vi "result_display.vi"(7 "note count":i32, 8 "lvl info":T1, 9 "score info":T2, 10 "timer":u32, 11 "new picture in":picture) -> (3 "new picture":picture)   [LabVIEW 2023]
uses:
  <vilib>/picture/picture.llb/Draw True-Color Pixmap.vi
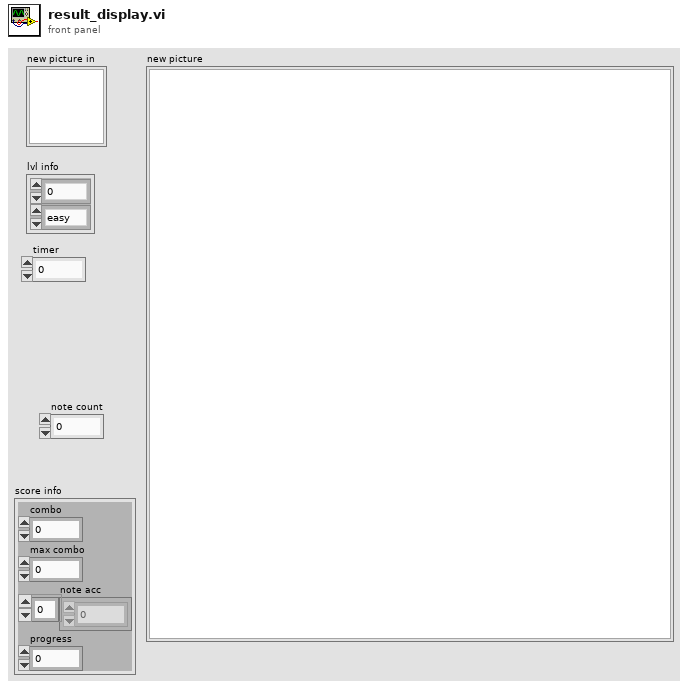
[diagram p1: front panel]
types:
  T1 = cluster{enum16{"0", "1"}, enum16{"easy", "hard"}}
  T2 = cluster{"combo":i32, "max combo":i32, "note acc":i32[], "progress":dbl}
  T3 = cluster{"horizontal":enum16{"left", "center", "right"}, "vertical":enum16{"top", "center", "bottom"}}
  T4 = cluster{"Font Name:":string, "Size":i16, "Strikeout?":bool, "Italic?":bool, "Underline?":bool, "Outline?":bool, "Shadow?":bool, "Bold?":bool}
  T5 = cluster{"Width":i16, "Style":enum32{"Solid", "Dash", "Dot", "DashDot", "DashDotDot"}}
  T6 = enum16{"User-specified Font", "Application Font", "System Font", "Dialog Font"}
  T7 = typedef "imagedata.ctl" = cluster{"image type":i32, "image depth":i32, "image":u8[], "mask":u8[], "colors":u32[], "Rectangle":cluster{"left":i16, "top":i16, "right":i16, "bottom":i16}}
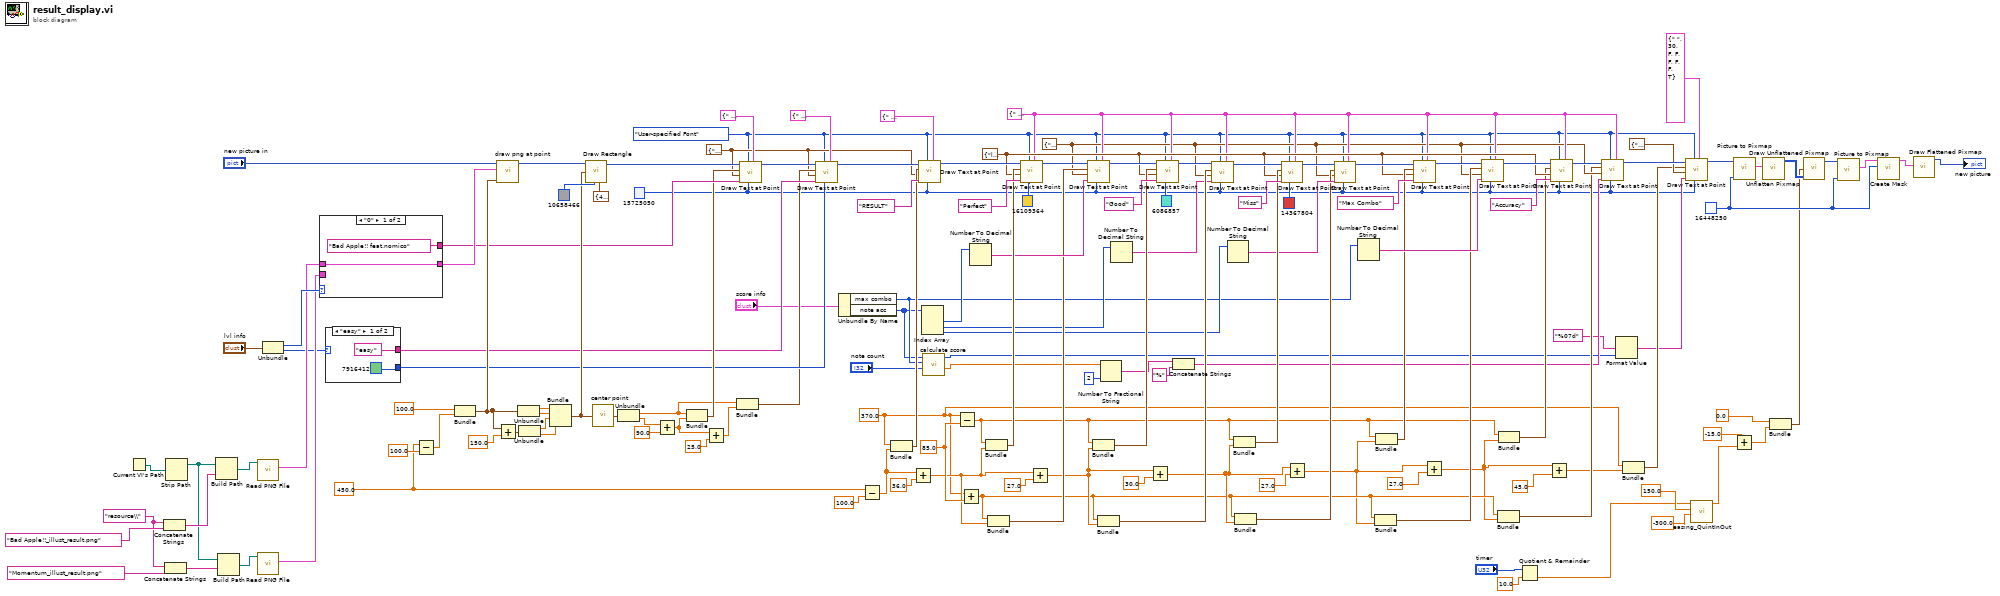
[diagram p0: block diagram]
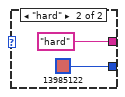
[diagram p2: hidden frame]
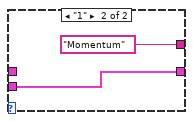
[diagram p3: hidden frame]
diagram:
  w11 = u32 16448250 ("color(black)")
  (unwired) 27.0
  w42 = T3 {"horizontal"=enum."right", "vertical"=enum."center"} ("alignment(left, top)")
  w50 = T3 {"horizontal"=enum."left", "vertical"=enum."center"} ("alignment(left, top)")
  w81 = 85.0
  w43 = T4 {"Font Name:"=" ", "Size"=20, "Strikeout?"=FALSE, "Italic?"=FALSE, "Underline?"=FALSE, "Outline?"=FALSE, "Shadow?"=FALSE, "Bold?"=TRUE} ("[user-specified font]")
  w125 = 450.0
  w20 = u32 15725050 ("text color(black)")
  w31 = 370.0
  w91 = T3 {"horizontal"=enum."center", "vertical"=enum."center"} ("alignment(left, top)")
  w27 = T6."User-specified Font" ("desired font(Application)")
  w142 = "resource\\"
  n1 = Current VI's Path() -> (path=w144:path)
  n2 = Concatenate Strings(w142, "Bad Apple!!_illust_result.png") -> (w140:string)
  n3 = Concatenate Strings(w142, "Momentum_illust_result.png") -> (w138:string)
  n4 = Strip Path(path=w144) -> (stripped path=w139:path)  [unwired: 1 out]
  n5 = Build Path(base path=w139, name or relative path=w140) -> (appended path=w137:path)
  n6 = Build Path(base path=w139, name or relative path=w138) -> (appended path=w136:path)
  n7 = call <vilib>:"Read PNG File.vi"("path to PNG file"=w137) -> ("image data"=w130:T7)  [unwired: 8 in, 2 out]
  n8 = call <vilib>:"Read PNG File.vi"("path to PNG file"=w136) -> ("image data"=w129:T7)  [unwired: 8 in, 2 out]
  n9 = Unbundle("lvl info") -> (w131:enum16{"0", "1"}, w104:enum16{"easy", "hard"})
  n10 = case shown="\"0\"" w131 {
    tunnel: w130 -> [w146 _]
    tunnel: w129 -> [_ w148]
    tunnel: [w146 w148] -> w127
    tunnel: ["Bad Apple!! feat.nomico" "Momentum"] -> w110
    frame "0" {
    }
    frame "1" {
    }
  }
  n11 = case shown="\"easy\"" w104 {
    tunnel: ["easy" "hard"] -> w100
    tunnel: [u32 7916412 ("color(black)") u32 13985122 ("color(black)")] -> w99
    frame "easy" {
    }
    frame "hard" {
    }
  }
  n12 = Subtract(x=w125, y=100.0) -> (x-y=w124:dbl)
  n13 = Bundle(100.0, w124) -> (w120:cluster{dbl, dbl})  [unwired: 1 in]
  n14 = call "draw png at point.vi"("top left point(0, 0)"=w120, "image data"=w127, "new picture in"="new picture in") -> ("new picture out"=w115:picture)  [unwired: 8 in]
  n15 = Add(x=w120, y=150.0) -> (x+y=w118:cluster{dbl, dbl})
  n16 = Unbundle(w120) -> (w122:dbl, w121:dbl)
  n17 = Unbundle(w118) -> (w117:dbl, w116:dbl)
  n18 = Bundle(w122, w121, w117, w116) -> (w112:cluster{dbl, dbl, dbl, dbl})  [unwired: 1 in]
  n19 = call <vilib>:"Draw Rectangle.vi"("picture"=w115, "rect"=w112, "color(black)"=u32 10658466, "pen"=T5 {"Width"=4, "Style"=enum."Solid"}) -> ("new picture"=w111:picture)  [unwired: 5 in]
  n20 = call "center point.vi"("border"=w112) -> ("center"=w108:cluster{dbl, dbl})  [unwired: 4 in]
  n21 = Unbundle(w108) -> (w98:dbl, w107:dbl)
  n22 = Add(x=w107, y=90.0) -> (x+y=w96:dbl)
  n23 = Bundle(w98, w96) -> (w105:cluster{dbl, dbl})  [unwired: 1 in]
  n24 = Add(x=w96, y=25.0) -> (x+y=w95:dbl)
  n25 = Bundle(w98, w95) -> (w94:cluster{dbl, dbl})  [unwired: 1 in]
  n26 = call <vilib>:"Draw Text at Point.vi"("[user-specified font]"=T4 {"Font Name:"=" ", "Size"=17, "Strikeout?"=FALSE, "Italic?"=FALSE, "Underline?"=FALSE, "Outline?"=FALSE, "Shadow?"=FALSE, "Bold?"=TRUE}, "text color(black)"=w20, "desired font(Application)"=w27, "text"=w110, "alignment(left, top)"=w91, "origin"=w105, "picture"=w111) -> ("new picture"=w103:picture)  [unwired: 3 in, 1 out]
  n27 = call <vilib>:"Draw Text at Point.vi"("[user-specified font]"=T4 {"Font Name:"=" ", "Size"=16, "Strikeout?"=FALSE, "Italic?"=FALSE, "Underline?"=FALSE, "Outline?"=FALSE, "Shadow?"=FALSE, "Bold?"=TRUE}, "text color(black)"=w99, "desired font(Application)"=w27, "text"=w100, "alignment(left, top)"=w91, "origin"=w94, "picture"=w103) -> ("new picture"=w101:picture)  [unwired: 3 in, 1 out]
  n28 = Unbundle By Name("score info") -> ("max combo"=w41:i32, "note acc"=w40:i32[])
  n29 = Subtract(x=w125, y=100.0) -> (x-y=w90:dbl)
  n30 = Bundle(w31, w90) -> (w133:cluster{dbl, dbl})  [unwired: 1 in]
  n31 = Add(x=w90, y=36.0) -> (x+y=w77:dbl)
  n32 = call <vilib>:"Draw Text at Point.vi"("[user-specified font]"=T4 {"Font Name:"=" ", "Size"=29, "Strikeout?"=FALSE, "Italic?"=FALSE, "Underline?"=FALSE, "Outline?"=FALSE, "Shadow?"=FALSE, "Bold?"=TRUE}, "text color(black)"=w20, "desired font(Application)"=w27, "text"="RESULT", "alignment(left, top)"=w91, "origin"=w133, "picture"=w101) -> ("new picture"=w93:picture)  [unwired: 3 in, 1 out]
  n33 = Index Array(array=w40) -> (element #1=w85:i32, element #2=w73:i32, element #3=w61:i32)  [unwired: 3 in]
  n34 = call "calculate score.vi"("note count"="note count", "max combo"=w41, "note acc"=w40) -> ("accuracy"=w36:dbl, "score"=w23:i32)  [unwired: 7 in]
  n35 = Subtract(x=w31, y=w81) -> (x-y=w49:dbl)
  n36 = Add(x=w31, y=w81) -> (x+y=w48:dbl)
  n37 = Number To Decimal String(number=w85) -> (decimal integer string=w84:string)  [unwired: 1 in]
  n38 = Bundle(w49, w77) -> (w88:cluster{dbl, dbl})  [unwired: 1 in]
  n39 = Bundle(w48, w77) -> (w82:cluster{dbl, dbl})  [unwired: 1 in]
  n40 = call <vilib>:"Draw Text at Point.vi"("[user-specified font]"=w43, "text color(black)"=u32 16109364, "desired font(Application)"=w27, "text"="Perfect", "alignment(left, top)"=w50, "origin"=w88, "picture"=w93) -> ("new picture"=w83:picture)  [unwired: 3 in, 1 out]
  n41 = Add(x=w77, y=27.0) -> (x+y=w66:dbl)
  n42 = call <vilib>:"Draw Text at Point.vi"("[user-specified font]"=w43, "text color(black)"=w20, "desired font(Application)"=w27, "text"=w84, "alignment(left, top)"=w42, "origin"=w82, "picture"=w83) -> ("new picture"=w80:picture)  [unwired: 3 in, 1 out]
  n43 = Bundle(w49, w66) -> (w75:cluster{dbl, dbl})  [unwired: 1 in]
  n44 = Bundle(w48, w66) -> (w74:cluster{dbl, dbl})  [unwired: 1 in]
  n45 = Number To Fractional String(number=w36, precision (6)=i16 2) -> (F-format string=w35:string)  [unwired: 2 in]
  n46 = Number To Decimal String(number=w73) -> (decimal integer string=w72:string)  [unwired: 1 in]
  n47 = Add(x=w66, y=30.0) -> (x+y=w55:dbl)
  n48 = call <vilib>:"Draw Text at Point.vi"("[user-specified font]"=w43, "text color(black)"=u32 6086857, "desired font(Application)"=w27, "text"="Good", "alignment(left, top)"=w50, "origin"=w75, "picture"=w80) -> ("new picture"=w71:picture)  [unwired: 3 in, 1 out]
  n49 = Concatenate Strings(w35, "%" ("string")) -> (w33:string)
  n50 = call <vilib>:"Draw Text at Point.vi"("[user-specified font]"=w43, "text color(black)"=w20, "desired font(Application)"=w27, "text"=w72, "alignment(left, top)"=w42, "origin"=w74, "picture"=w71) -> ("new picture"=w70:picture)  [unwired: 3 in, 1 out]
  n51 = Number To Decimal String(number=w61) -> (decimal integer string=w64:string)  [unwired: 1 in]
  n52 = Bundle(w49, w55) -> (w65:cluster{dbl, dbl})  [unwired: 1 in]
  n53 = Bundle(w48, w55) -> (w62:cluster{dbl, dbl})  [unwired: 1 in]
  n54 = call <vilib>:"Draw Text at Point.vi"("[user-specified font]"=w43, "text color(black)"=u32 14367804, "desired font(Application)"=w27, "text"="Miss", "alignment(left, top)"=w50, "origin"=w65, "picture"=w70) -> ("new picture"=w63:picture)  [unwired: 3 in, 1 out]
  n55 = Add(x=w55, y=27.0) -> (x+y=w47:dbl)
  n56 = call <vilib>:"Draw Text at Point.vi"("[user-specified font]"=w43, "text color(black)"=w20, "desired font(Application)"=w27, "text"=w64, "alignment(left, top)"=w42, "origin"=w62, "picture"=w63) -> ("new picture"=w60:picture)  [unwired: 3 in, 1 out]
  n57 = Number To Decimal String(number=w41) -> (decimal integer string=w57:string)  [unwired: 1 in]
  n58 = Bundle(w48, w47) -> (w53:cluster{dbl, dbl})  [unwired: 1 in]
  n59 = Bundle(w49, w47) -> (w54:cluster{dbl, dbl})  [unwired: 1 in]
  n60 = call <vilib>:"Draw Text at Point.vi"("[user-specified font]"=w43, "text color(black)"=w20, "desired font(Application)"=w27, "text"="Max Combo", "alignment(left, top)"=w50, "origin"=w54, "picture"=w60) -> ("new picture"=w58:picture)  [unwired: 3 in, 1 out]
  n61 = Add(x=w47, y=27.0) -> (x+y=w29:dbl)
  n62 = call <vilib>:"Draw Text at Point.vi"("[user-specified font]"=w43, "text color(black)"=w20, "desired font(Application)"=w27, "text"=w57, "alignment(left, top)"=w42, "origin"=w53, "picture"=w58) -> ("new picture"=w52:picture)  [unwired: 3 in, 1 out]
  n63 = Bundle(w48, w29) -> (w38:cluster{dbl, dbl})  [unwired: 1 in]
  n64 = Bundle(w49, w29) -> (w45:cluster{dbl, dbl})  [unwired: 1 in]
  n65 = Quotient & Remainder(x="timer", y=10.0 ("interval (10 ms)")) -> (floor(x/y)=w4:dbl)  [unwired: 1 out]
  n66 = Add(x=w29, y=45.0) -> (x+y=w28:dbl)
  n67 = call <vilib>:"Draw Text at Point.vi"("[user-specified font]"=w43, "text color(black)"=w20, "desired font(Application)"=w27, "text"="Accuracy", "alignment(left, top)"=w50, "origin"=w45, "picture"=w52) -> ("new picture"=w44:picture)  [unwired: 3 in, 1 out]
  n68 = call <vilib>:"Draw Text at Point.vi"("[user-specified font]"=w43, "text color(black)"=w20, "desired font(Application)"=w27, "text"=w33, "alignment(left, top)"=w42, "origin"=w38, "picture"=w44) -> ("new picture"=w32:picture)  [unwired: 3 in, 1 out]
  n69 = Format Value(format string="%07d", value (0)=w23) -> (output string=w21:string)  [unwired: 1 in]
  n70 = Bundle(w31, w28) -> (w24:cluster{dbl, dbl})  [unwired: 1 in]
  n71 = call <vilib>:"Draw Text at Point.vi"("[user-specified font]"=T4 {"Font Name:"=" ", "Size"=30, "Strikeout?"=FALSE, "Italic?"=FALSE, "Underline?"=FALSE, "Outline?"=FALSE, "Shadow?"=FALSE, "Bold?"=TRUE}, "text color(black)"=w20, "desired font(Application)"=w27, "text"=w21, "alignment(left, top)"=T3 {"horizontal"=enum."center", "vertical"=enum."center"}, "origin"=w24, "picture"=w32) -> ("new picture"=w16:picture)  [unwired: 3 in, 1 out]
  n72 = call "easing_QuintInOut.vi"("distance"=-300.0, "interval (10 ms)"=150.0, "time"=w4) -> ("current position"=w2:dbl)  [unwired: 8 in]
  n73 = Add(x=-15.0 ("interval (10 ms)"), y=w2) -> (x+y=w3:dbl)
  n74 = call <vilib>:"Picture to Pixmap.vi"("Background Color"=w11, "picture"=w16) -> ("image data"=w15:T7)  [unwired: 8 in, 1 out]
  n75 = call <vilib>:"Unflatten Pixmap.vi"("image data"=w15) -> ("24-bit pixmap"=w14:u32[][])  [unwired: 4 in, 6 out]
  n76 = Bundle("interval (10 ms)"=0.0, w3) -> (w7:cluster{"interval (10 ms)":dbl, dbl})  [unwired: 1 in]
  n77 = call-poly <vilib>:"Draw Unflattened Pixmap.vi"("top left point(0, 0)"=w7, "data (RGB format)"=w14) -> ("new picture"=w13:picture)  [unwired: 7 in]
  n78 = call <vilib>:"Picture to Pixmap.vi"("Background Color"=w11, "picture"=w13) -> ("image data"=w12:T7)  [unwired: 8 in, 1 out]
  n79 = call <vilib>:"Create Mask.vi"("Mask Color (Black)"=w11, "image data"=w12) -> ("image data"=w10:T7)  [unwired: 9 in]
  n80 = call <vilib>:"Draw Flattened Pixmap.vi"("image data"=w10) -> ("new picture"=→"new picture":picture)  [unwired: 8 in]
